vi "tool call.vi"(8 "error in":errorcluster, 10 "id in":i32, 11 "message json":string) -> (0 "error out":errorcluster, 3 "response":string)   [LabVIEW 2025, in "MCP Server.lvlib"]
uses:
  MCP Server.lvlib
  affbca46-cbce-409b-bfea-a62add01a465.vi
  <vilib>/JDP Science/JSONtext/Next JSON Value.vi
  <vilib>/JDP Science/JSONtext/String Subset.vi
  <vilib>/JDP Science/JSONtext/Parsing/Advance past next JSON Value (inlined COPY).vi
  <vilib>/JDP Science/JSONtext/Parsing/Advance past whitespace.vi
  <vilib>/JDP Science/JSONtext/Parsing/Advance past String.vi
  <vilib>/JDP Science/JSONtext/Parsing/Advance past Number.vi
  <vilib>/JDP Science/JSONtext/Parsing/Advance past Line Ending.vi
  <vilib>/JDP Science/JSONtext/Parsing/Parse Full Path or Item Name.vi
  <vilib>/JDP Science/JSONtext/Parsing/Advance past Array.vi
  <vilib>/JDP Science/JSONtext/Parsing/Advance past Object.vi
  <vilib>/JDP Science/JSONtext/support/Error Cluster From Code.vi
  <vilib>/JDP Science/JSONtext/Offset/Find Item Locations by Path.vi
  <vilib>/JDP Science/JSONtext/JSON text to Variant.vi
  <vilib>/JDP Science/JSONtext/LVClass Serializer/JSONtext LVClass Serializer.lvclass
  <vilib>/JDP Science/JSONtext/JSONtext.lvlib
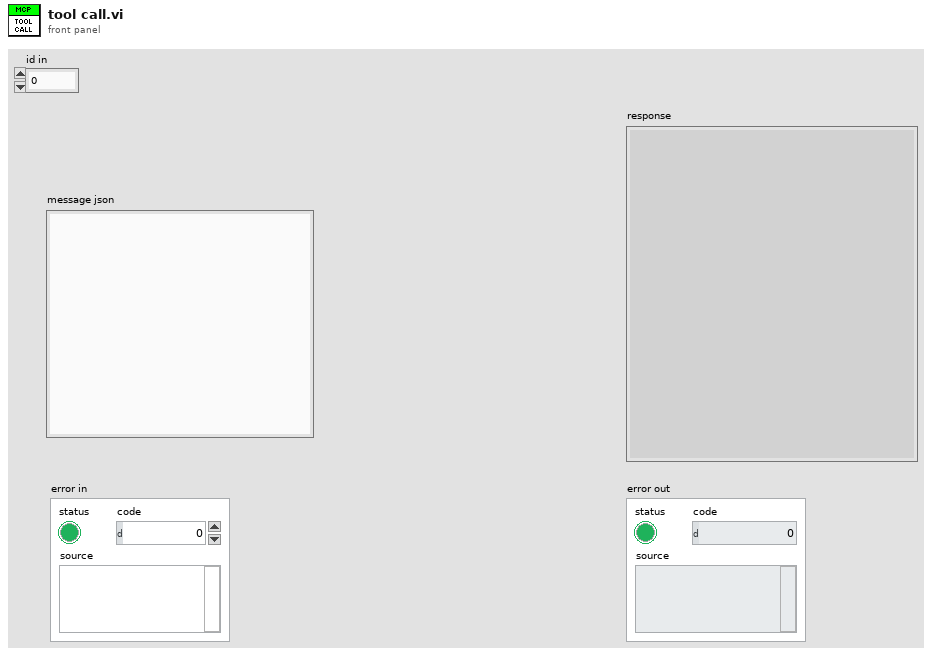
[diagram p1: front panel]
types:
  T1 = typedef "MCP Server.lvlib/Tool Data.ctl" = cluster{"Name":string, "Description":string, "Ignored":string[], "inputs":T2[], "outputs":T3[], "VI Refnum":refnum<vi>}
  T2 = typedef "MCP Server.lvlib/Input Parameter.ctl" = cluster{"name":string, "type":string, "description":string, "required":bool, "raw name":string}
  T3 = typedef "MCP Server.lvlib/Output Parameter.ctl" = cluster{"name":string, "description":string, "type":string, "raw name":string}
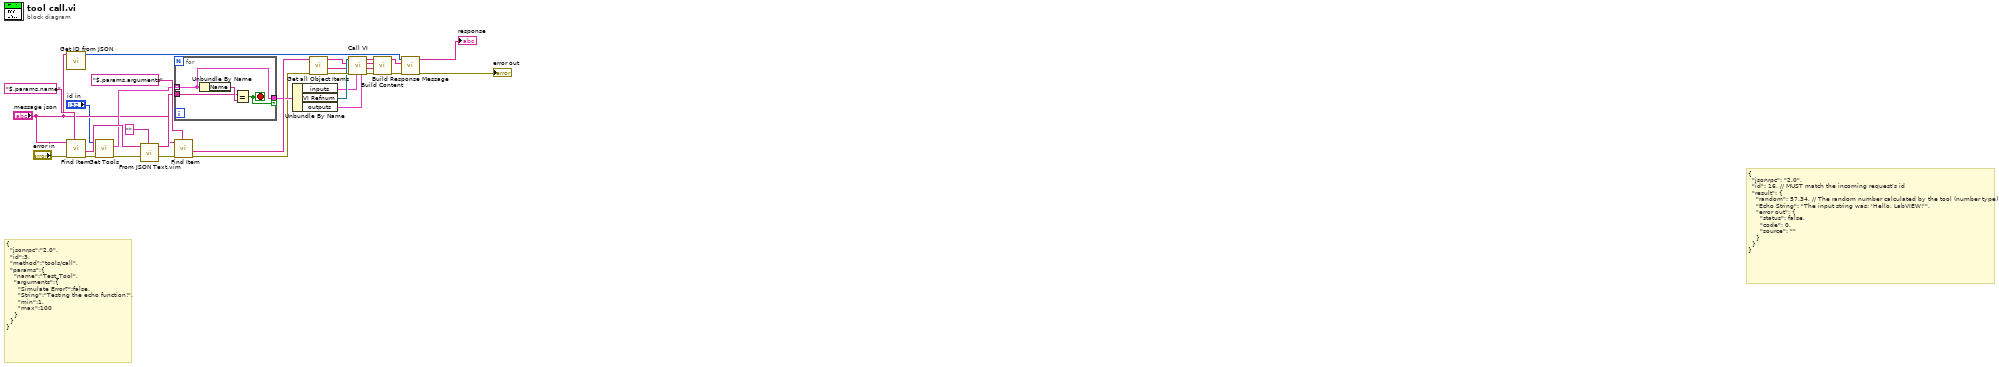
[diagram p0: block diagram]
diagram:
  # "{\n  \"jsonrpc\": \"2.0\",\n  \"id\": 16, // MUST match the incoming request's id\n  \"result\": {\n    \"random\": 57.34, // The random number calculated by the tool (number type)\n    \"Echo String\": \"The input string was: 'Hello, LabVIEW!'\",\n    \"error out\": {\n      \"status\": false,\n      \"code\": 0,\n      \"source\": \"\"\n    }\n  }\n}"
  # "{\n  \"jsonrpc\":\"2.0\",\n  \"id\":3,\n  \"method\":\"tools/call\",\n  \"params\":{\n    \"name\":\"Test_Tool\",\n    \"arguments\":{\n      \"Simulate Error?\":false,\n      \"String\":\"Testing the echo function!\",\n      \"min\":1,\n      \"max\":100\n    }\n  }\n}"
  n1 = call "Get ID from JSON.vi"("message json"="message json") -> ("Data out"=w26:i32)  [unwired: 10 in]
  n2 = call <vilib>:"Find Item.vi"("$Path or Item Name"="$.params.name", "error in (no error)"="error in", "JSON"="message json") -> ("error out"=w12:errorcluster, "<JSON>"=w23:string)  [unwired: 5 in, 2 out]
  n3 = call "Get Tools.vi"("error in (no error)"=w12, "server id in"="id in") -> ("error out"=w13:errorcluster, "Tools"=w20:T1[])  [unwired: 7 in, 1 out]
  n4 = call "From JSON Text.vim"("Data Type and Default Value"="" ("$Path or Item Name"), "error in (no error)"=w13, "JSON"=w23) -> ("error out"=w11:errorcluster, "Data out"=w22:string)  [unwired: 7 in]
  n5 = for {
    tunnel: w20 -> [w32] mode=indexing
    tunnel: w22 -> [w33]
    tunnel: [w32] -> w19 if=w31
    stop <- w31 stop-if-true
    n6 = Unbundle By Name(w32) -> ("Name"=w34:string)
    n7 = Equal?(x=w33, y=w34) -> (x = y?=w31:bool)
  }
  n8 = call <vilib>:"Find Item.vi"("$Path or Item Name"="$.params.arguments", "error in (no error)"=w11, "JSON"="message json") -> ("error out"=w10:errorcluster, "<JSON>"=w29:string)  [unwired: 5 in, 2 out]
  n9 = Unbundle By Name(w19) -> ("inputs"=w3:T2[], "VI Refnum"=w6:refnum<vi>, "outputs"=w2:T3[])
  n10 = call <vilib>:"Get all Object Items.vi"("error in (no error)"=w10, "JSON"=w29) -> ("error out"=w9:errorcluster, "<JSON>"=w4:string[], "Item Names"=w5:string[])  [unwired: 6 in, 1 out]
  n11 = call "Call VI.vi"("output info"=w2, "input info"=w3, "error in (no error)"=w9, "Input Values"=w4, "Input Names"=w5, "VI in"=w6) -> ("error out"=w7:errorcluster, "output values"=w28:string[], "output names"=w27:string[], "pictures"=w16:string[])  [unwired: 2 in]
  n12 = call "Build Content.vi"("error in (no error)"=w7, "values"=w28, "names"=w27, "pictures"=w16) -> ("error out"=w1:errorcluster, "<JSON>"=w25:string)  [unwired: 6 in]
  n13 = call "Build Response Message.vi"("error in (no error)"=w1, "Result content"=w25, "message id in"=w26) -> ("error out"=→"error out":errorcluster, "MCP message out"=→"response":string)  [unwired: 7 in]
